vi "FP forebrain ACT.vi"(2 "error in":errorcluster, 3 "local Steering\nangle":dbl=-135.0 format="%#_13g", 4 "Behaviors in":T1) -> (0 "error out":errorcluster, 1 "Forebrain ACT":dbl[](array[numeric]))   [LabVIEW 2014]
panel:
  out "Forebrain ACT Graph":cluster{dbl, dbl, dbl[]}(graph)
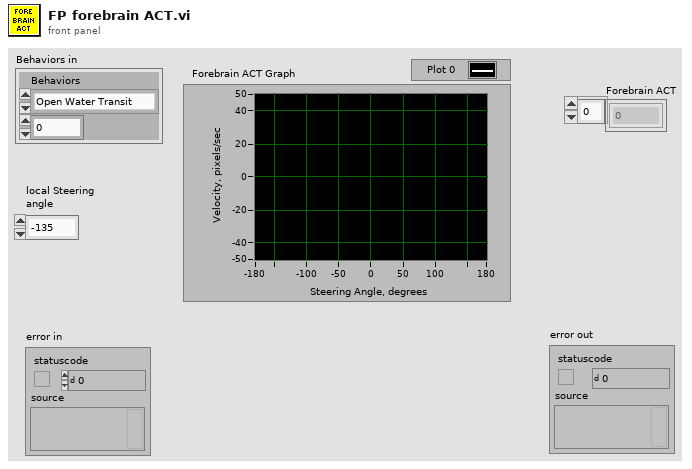
[diagram p1: front panel]
types:
  T1 = cluster{"Behaviors":enum16{"Open Water Transit", "P-Wall Follow", "S-Wall Follow", "Dock"}, dbl}
  T2 = enum16{"Open Water Transit", "P-Wall Follow", "S-Wall Follow", "Dock"}
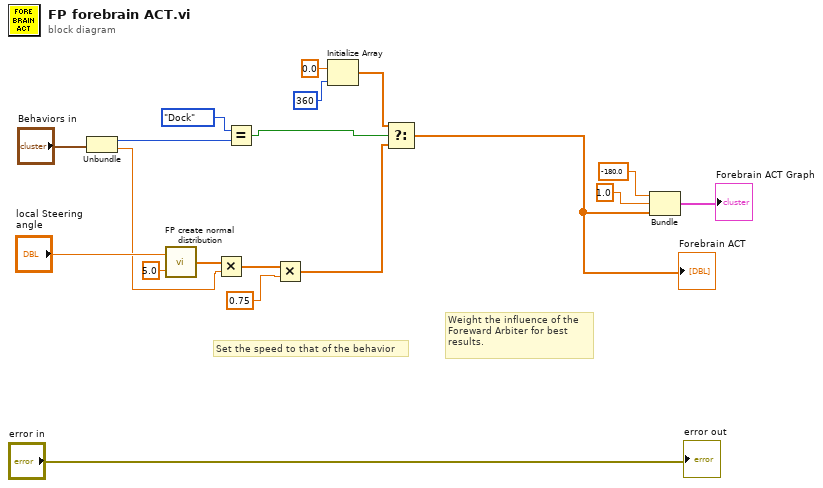
[diagram p0: block diagram]
diagram:
  # "Weight the influence of the\nForeward Arbiter for best\nresults."
  # "Set the speed to that of the behavior"
  n1 = Unbundle("Behaviors in") -> ("Behaviors"=w2:T2, w11:dbl)
  n2 = call "FP create normal distribution.vi"("std (Normal)"=5.0, "mean"="local Steering\nangle") -> ("ACT array"=w17:dbl[])
  n3 = Multiply(x=w17, y=w11) -> (x*y=w10:dbl[])
  n4 = Equal?(x=T2."Dock", y=w2) -> (x = y?=w1:bool)
  n5 = Multiply(x=w10, y=0.75 ("Arbiter weight")) -> (x*y=w7:dbl[])
  n6 = Initialize Array(0.0 ("element"), 360 ("dimension size")) -> (w3:dbl[])
  n7 = Select(t=w3, s=w1, f=w7) -> (s? t:f=w6:dbl[])
  "Forebrain ACT" <- w6
  n8 = Bundle(-180.0, 1.0, w6) -> (→"Forebrain ACT Graph":cluster{dbl, dbl, dbl[]})  [unwired: 1 in]
  "error out" <- "error in"
